vi "Pack Message.vi"(8 "error in (no error)":errorcluster, 11 "Car Position Changed in":refnum<class "Car Position Changed.lvclass">) -> (0 "error out":errorcluster, 1 "Packed Message":string, 2 "Message Name":string, 3 "Car Position Changed out":refnum<class "Car Position Changed.lvclass">)   [LabVIEW 2016, in "CLD Exam - Car Wash.lvlib" / "Car Position Changed.lvclass"]
uses:
  Car Position Changed.lvclass
  D:/Repos/Stream/software/Mediator/Classes/Message Interface/Message Interface.lvclass
  Car Position Changed.lvclass/Car Position Changed.ctl
  Mediator/Classes/Message Interface/Message Interface.lvclass
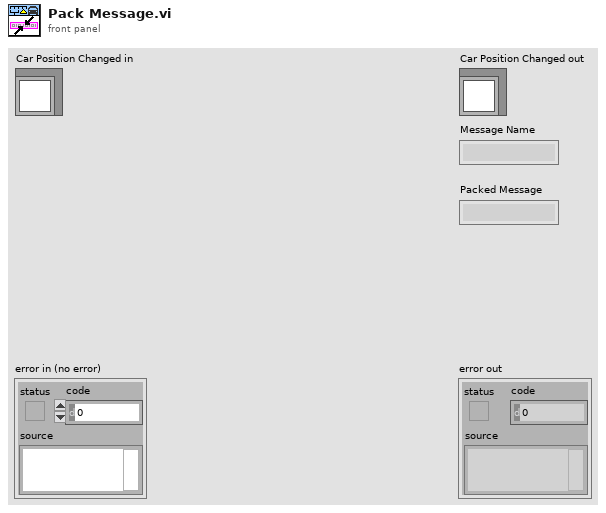
[diagram p1: front panel]
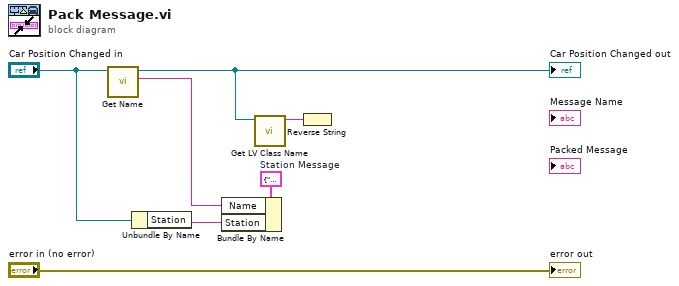
[diagram p0: block diagram]
diagram:
  w6 = cluster{"Station":string, "Name":string} {"Station"="", "Name"=""}  # Station Message
  n1 = call "Get Name.vi"("Message Interface in"="Car Position Changed in") -> ("Name"=w4:string, "Message Interface out"=w3:refnum<class "Car Position Changed.lvclass">)  [unwired: 8 in, 1 out]
  "Car Position Changed out" <- w3
  n2 = Unbundle By Name("Car Position Changed in") -> ("Station"=w5:string)
  n3 = Bundle By Name(cluster=w6, "Name"=w4, "Station"=w5) -> ()  [unwired: 1 out]
  n4 = call <vilib>:"Get LV Class Name.vi"("object"=w3) -> ("class name"=w2:string)  [unwired: 9 in, 1 out]
  n5 = Reverse String(1:w2) -> ()  [unwired: 1 out]
  "error out" <- "error in (no error)"
